vi "ex_UnflattenDescriptionString.vi"(0 "Description":string, 1 "Comment":string) -> (2 "Description Out":string, 3 "Comment Out":string, 4 "DAQmx Task":T1)   [LabVIEW 2020]
uses:
  express shared/ex_EditUserDefinedProperties/ex_userdefproperties.ctl
  express shared/ExFile.llb/ex_userDefProperty.ctl
  express shared/ex_EditUserDefinedProperties/usiDataType.ctl
  express shared/ExFile.llb/ex_propertySource.ctl
panel:
  in  "DAQmxTask":T1
  in  "Description Cluster":T5
  in  "user-def properties":T1
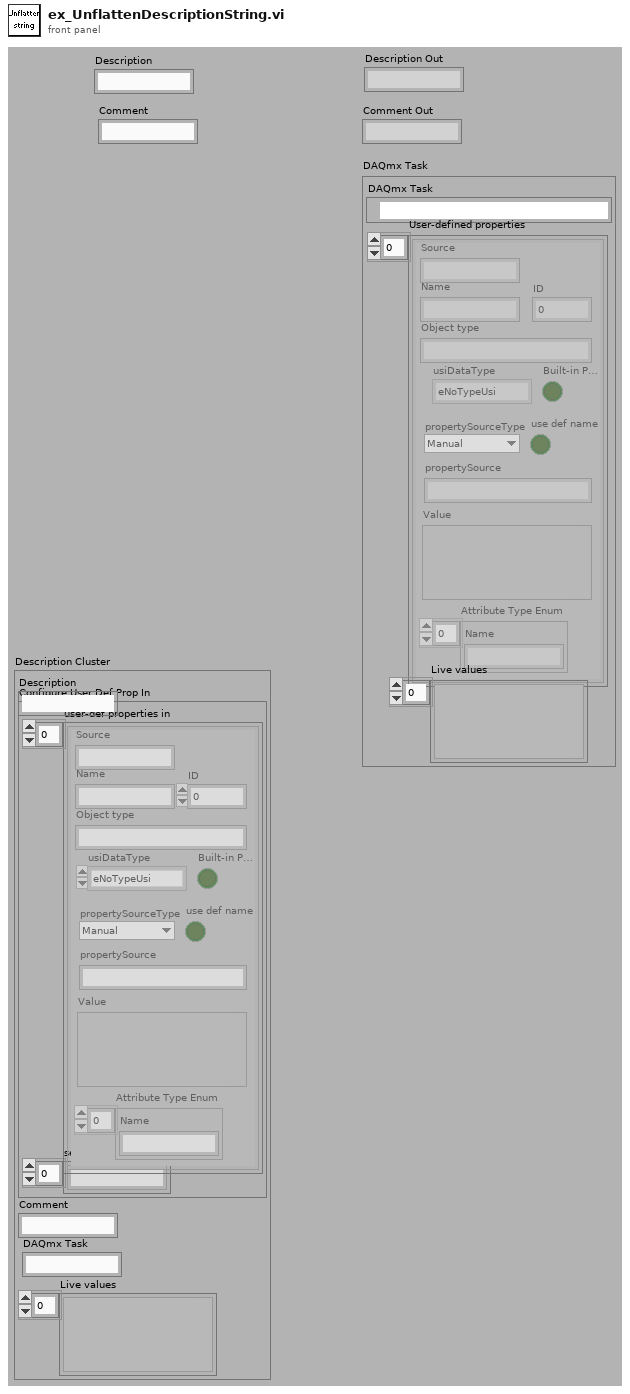
[diagram p1: front panel]
types:
  T1 = typedef "ex_userdefproperties.ctl" = cluster{"DAQmx Task":refnum<k21>, "User-defined properties":T2[], "Live values":variant[]}
  T2 = typedef "ex_userDefProperty.ctl" = cluster{"Name":string, "Object type":string, "usiDataType":T3, "propertySourceType":T4, "propertySource":string, "Value":variant, "ID":i32, "use def name":bool, "Source":string, "Built-in Prop":bool, "Attribute Type Enum":string[]}
  T3 = typedef "usiDataType.ctl" = enum16{"eNoTypeUsi", "eInt8Usi", "eInt16Usi", "eInt32Usi", "eInt64Usi", "eUInt8Usi", "eUInt16Usi", "eUInt32Usi", "eUInt64Usi", "eFloat32Usi", "eFloat64Usi", "- 0", "- 1", "- 2", "- 3", "- 4", "- 5", "- 6", "- 7", "- 8", "- 9", "eString8Usi", "eString16Usi", "eStringUsi", "eEnumUsi", "- 10", "- 11", "- 12", "- 13", "- 14", "eTimeUsi", "- 15", "- 16", "- 17", "- 18", "- 19", "- 20", "- 21", "- 22", "- 23", "eInstanceUsi", "eStoreUsi"}
  T4 = typedef "ex_propertySource.ctl" = enum16{"Manual", "System", "DAQmx Channel", "Terminal", "Ignore"}
  T5 = cluster{"Description":string, "Configure User Def Prop In":cluster{"user-def properties in":T2[], "selected nodes in":string[]}, "Comment":string, "DAQmx Task":string, "Live values":variant[]}
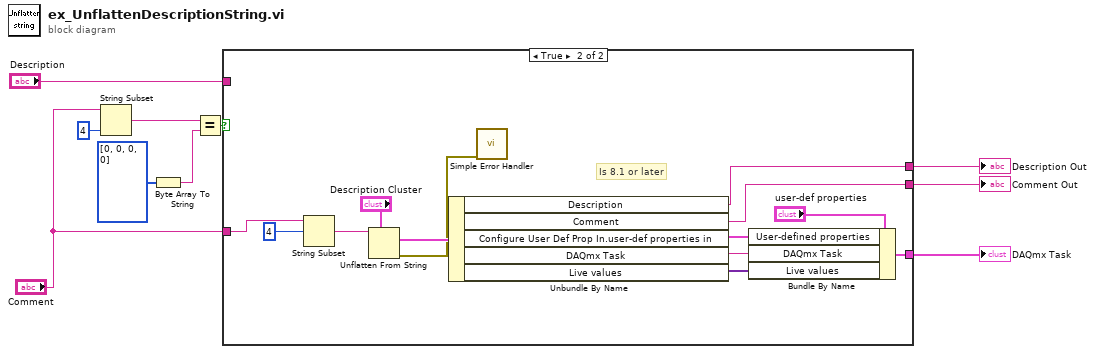
[diagram p0: block diagram]
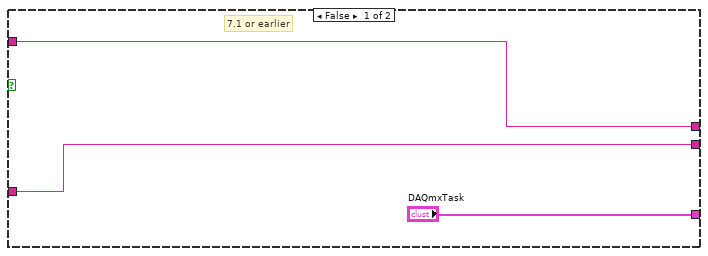
[diagram p2: hidden frame]
diagram:
  n1 = String Subset(string="Comment", length (rest)=4 ("length (rest)")) -> (substring=w9:string)  [unwired: 1 out]
  n2 = Byte Array To String(unsigned byte array=u8[] [0, 0, 0, 0]) -> (string=w2:string)
  n3 = Equal?(x=w9, y=w2) -> (x = y?=w10:bool)
  n4 = case shown="True" w10 {
    tunnel: "Comment" -> [w12 w18]
    tunnel: [w13 w21] -> w3
    tunnel: [w12 w20] -> w4
    tunnel: ["DAQmxTask" w22] -> w5
    tunnel: "Description" -> [w13 _]
    frame False {
      # "7.1 or earlier"
    }
    frame True {
      # "Is 8.1 or later"
      n5 = String Subset(string=w18, offset (0)=4) -> (substring=w16:string)  [unwired: 1 out]
      n6 = Unflatten From String(type="Description Cluster", binary string=w16) -> (value=w23:T5, error out=w15:errorcluster)  [unwired: 1 in, 3 out]
      n7 = Unbundle By Name(w23) -> ("Description"=w21:string, "Comment"=w20:string, "Configure User Def Prop In.user-def properties in"=w14:T2[], "DAQmx Task"=w25:string, "Live values"=w19:variant[])
      n8 = call "Simple Error Handler.vi"("error in (no error)"=w15) -> ()  [unwired: 1 in, 8 out]
      n9 = Bundle By Name(cluster="user-def properties", "User-defined properties"=w14, "DAQmx Task"=w25, "Live values"=w19) -> (w22:T1)
    }
  }
  "DAQmx Task" <- w5
  "Comment Out" <- w4
  "Description Out" <- w3
